vi "Delete Item from LVClass.vi"(7 "Item Type":string="VI", 8 "error in (no error)":errorcluster, 10 "Item name":string, 11 "LVClassLibrary in":refnum<vi>) -> (0 "error out":errorcluster, 2 "Deleted ?":bool, 3 "LVClassLibrary out":refnum<vi>)   [LabVIEW 2019, in "gRPC Scripting Tools.lvlib"]
uses:
  gRPC Scripting Tools.lvlib
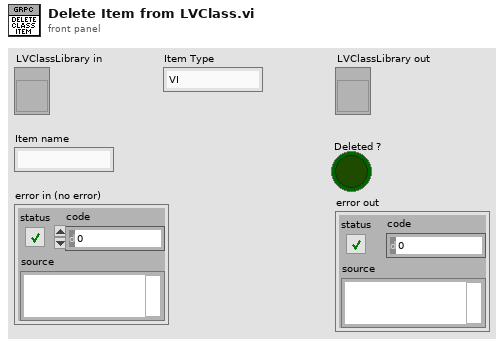
[diagram p1: front panel]
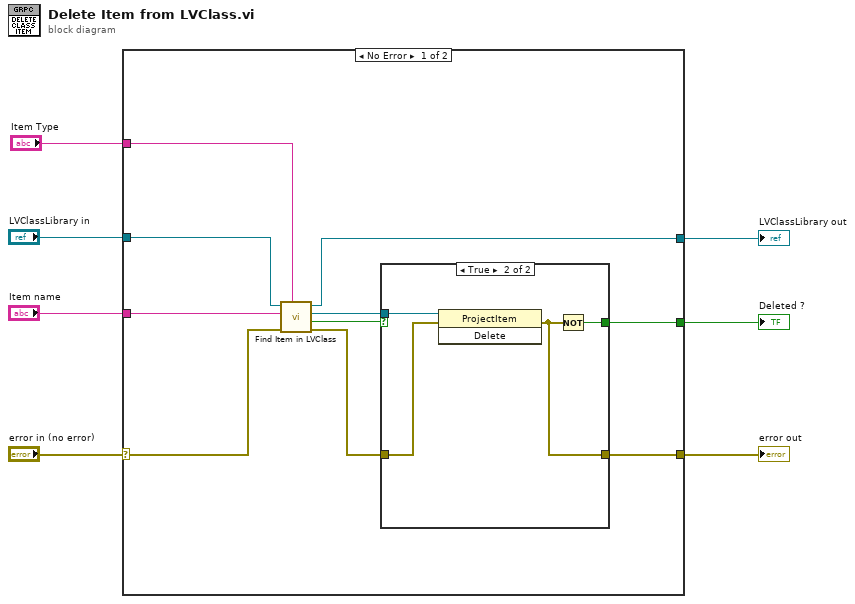
[diagram p0: block diagram]
diagram:
  n1 = case shown="No Error" "error in (no error)" {
    selector: "error in (no error)" -> [w10 w24]
    tunnel: [w17 w23] -> w7
    tunnel: "Item name" -> [w16 _]
    tunnel: "LVClassLibrary in" -> [w15 w23]
    tunnel: "Item Type" -> [w14 _]
    tunnel: [w9 w24] -> w2
    tunnel: [w8 _] -> w1
    frame No Error {
      n2 = call "Find Item in LVClass.vi"("Item Type"=w14, "error in (no error)"=w10, "Item Name"=w16, "Class Item in"=w15) -> ("error out"=w11:errorcluster, "Found?"=w13:bool, "Project Item (Class Item)"=w12:refnum<vi>, "Class Item out"=w17:refnum<vi>)  [unwired: 4 in]
      n3 = case shown="True" w13 {
        tunnel: w12 -> [_ w22]
        tunnel: w11 -> [w18 w21]
        tunnel: [w18 w20] -> w9
        tunnel: [_ w19] -> w8
        frame False {
        }
        frame True {
          n4 = invoke class="ProjectItem" method="Delete"(reference=w22, error in=w21) -> (error out=w20:errorcluster)  [unwired: 1 in, 2 out]
          n5 = Not(x=w20) -> (.not. x?=w19:bool)
        }
      }
    }
    frame Error {
    }
  }
  "LVClassLibrary out" <- w7
  "error out" <- w2
  "Deleted ?" <- w1
